vi "getName.vi"(8 "error in (no error)":errorcluster, 11 "xmlNode.lvclass in":refnum<class "xmlNode.lvclass">) -> (0 "error out":errorcluster, 2 "name":string, 3 "xmlNode.lvclass out":refnum<class "xmlNode.lvclass">)   [LabVIEW 2009, in "Tools.lvlib" / "xml.lvlib" / "xmlNode.lvclass"]
doc: "Gets the name of the xml node\nGets \"name\" in this example\n\n<\"name\">\n <child xml element 1> value </child xml element 1>\n <child xml element 2> value </child xml element 2>\n</\"name\">"
uses:
  xmlNode.lvclass
  xmlNode.lvclass/xmlNode.ctl
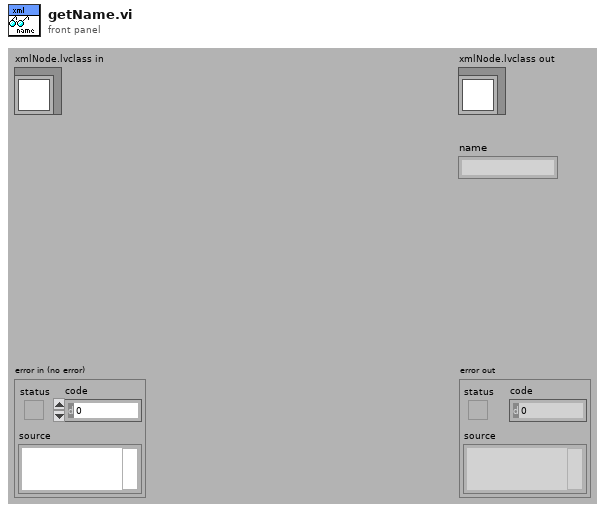
[diagram p1: front panel]
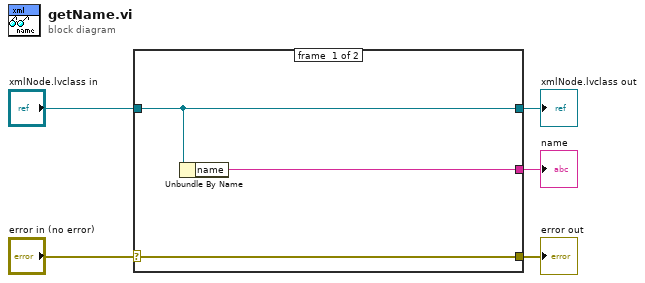
[diagram p0: block diagram]
diagram:
  n1 = case shown="No Error" "error in (no error)" {
    selector: "error in (no error)" -> [w8 w9]
    tunnel: [w8 w9] -> w4
    tunnel: [w7 w10] -> w2
    tunnel: "xmlNode.lvclass in" -> [w7 w10]
    tunnel: [w6 _] -> w1
    frame #0 {
      n2 = Unbundle By Name(w7) -> ("name"=w6:string)
    }
    frame #1 {
    }
  }
  "error out" <- w4
  "xmlNode.lvclass out" <- w2
  "name" <- w1
